vi "Bitcrush.vi"(0 "IN":dbl[](array[numeric]), 1 "Bitcrusher":dbl) -> (6 "OUT":dbl[](array[numeric]))   [LabVIEW 2025]
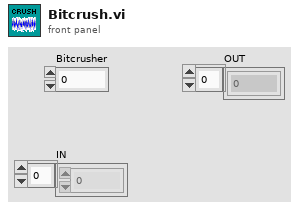
[diagram p1: front panel]
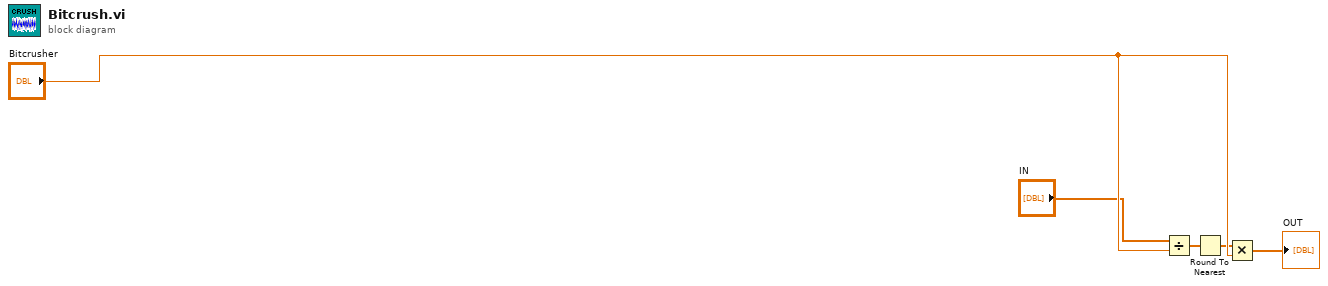
[diagram p0: block diagram]
diagram:
  n1 = Divide(x="IN", y="Bitcrusher") -> (x/y=w2:dbl[])
  n2 = Round To Nearest(number=w2) -> (nearest integer value=w3:dbl[])
  n3 = Multiply(x=w3, y="Bitcrusher") -> (x*y=→"OUT":dbl[])
